vi "Read ini file.vi"(6 "INI FileFullName":T1="Config.ini", 8 "error in (no error)":errorcluster, 10 "VariableName":string, 11 "section":string) -> (0 "error out":errorcluster, 1 "Boolean":bool, 2 "String value":string, 3 "DBL Value":dbl format="%#_6f", 4 "file path":path, 5 "Int Value":i32)   [LabVIEW 2021, in "File RW.lvlib"]
uses:
  <userlib>/John_Lib/File/File RW.lvlib
  <userlib>/John_Lib/File/FileName.ctl
  <vilib>/Utility/config.llb/Read Key (String).vi
  <vilib>/Utility/config.llb/NI_LVConfig.lvlib
  <userlib>/John_Lib/TopPath/TopPath.lvlib
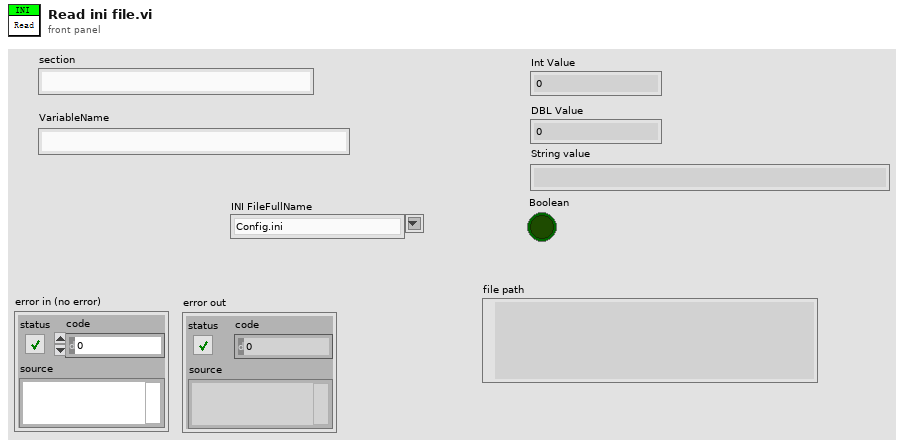
[diagram p1: front panel]
types:
  T1 = typedef "File RW.lvlib/FileName.ctl" = string
  T2 = typedef "NI_LVConfig.lvlib/Config Data RefNum.ctl" = refnum<k1>
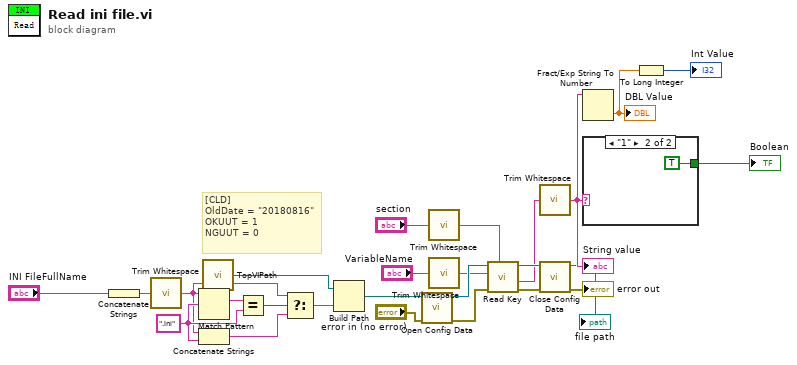
[diagram p0: block diagram]
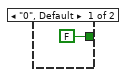
[diagram p2: hidden frame]
diagram:
  w11 = ".ini" ("regular expression")
  # "[CLD]\nOldDate = \"20180816\"\nOKUUT = 1    \nNGUUT = 0"
  n1 = Concatenate Strings("INI FileFullName") -> (w3:string)
  n2 = call <vilib>:"Trim Whitespace.vi"("string"=w3) -> ("trimmed string"=w6:string)  [unwired: 1 in]
  n3 = Match Pattern(string=w6, regular expression=w11) -> (match substring=w9:string)  [unwired: 1 in, 3 out]
  n4 = Concatenate Strings(w6, w11) -> (w12:string)
  n5 = call <userlib>:"TopVIPath.vi"() -> ("ConfigFile path"=w2:path)  [unwired: 2 out]
  n6 = Equal?(x=w9, y=w11) -> (x = y?=w10:bool)
  n7 = Select(t=w6, s=w10, f=w12) -> (s? t:f=w8:string)
  n8 = Build Path(base path=w2, name or relative path=w8) -> (appended path=w17:path)
  n9 = call <vilib>:"Open Config Data.vi"("error in (no error)"="error in (no error)", "configuration file path"=w17) -> ("error out"=w25:errorcluster, "refnum"=w26:T2)  [unwired: 7 in, 1 out]
  n10 = call <vilib>:"Trim Whitespace.vi"("string"="section") -> ("trimmed string"=w7:string)  [unwired: 1 in]
  n11 = call <vilib>:"Trim Whitespace.vi"("string"="VariableName") -> ("trimmed string"=w18:string)  [unwired: 1 in]
  n12 = call-poly <vilib>:"Read Key.vi"("section"=w7, "error in (no error)"=w25, "key"=w18, "refnum"=w26) -> ("error out"=w20:errorcluster, "value"=w15:string, "refnum out"=w19:T2)  [unwired: 4 in, 1 out]
  n13 = call <vilib>:"Trim Whitespace.vi"("string"=w15) -> ("trimmed string"=w5:string)  [unwired: 1 in]
  "String value" <- w5
  n14 = call <vilib>:"Close Config Data.vi"("error in (no error)"=w20, "refnum"=w19) -> ("error out"=→"error out":errorcluster, "file path"=→"file path":path)  [unwired: 8 in]
  n15 = Fract/Exp String To Number(string=w5) -> (number=w14:dbl)  [unwired: 3 in, 1 out]
  "DBL Value" <- w14
  n16 = case shown="\"1\"" w5 {
    tunnel: [FALSE ("Boolean") TRUE ("Boolean")] -> w16
    frame "0", Default {
    }
    frame "1" {
    }
  }
  "Boolean" <- w16
  n17 = To Long Integer(number=w14) -> (32bit integer=→"Int Value":i32)
